vi "Resize and Align.vi"(9 "number of channels":i32, 10 "Refnums for Resizing and Alignment":T4, 11 "State in":T1={"Graph Visible Items"={"Plot Legend"=FALSE, "Scale Legend"=FALSE, "Graph Palette"=FALSE, "Cursor Legend"=FALSE, "X Scrollbar"=FALSE}, "View Table"=FALSE, "Table Visible Items"={"Vertical Scrollbar"=FALSE, "Horizontal Scrollbar"=FALSE, "Row Headers"=FALSE, "Column Headers"=FALSE, "Vertical Lines"=FALSE, "Horizontal Lines"=FALSE}, "Header Font"={"Font Name"="", "Size"=0, "Bold"=FALSE, "Italic"=FALSE, "Underline"=FALSE, "Strikeout"=FALSE, "Color"=0}, "Cell Font"={"Font Name"="", "Size"=0, "Bold"=FALSE, "Italic"=FALSE, "Underline"=FALSE, "Strikeout"=FALSE, "Color"=0}, "Description and Tip..."={"Description"="", "Tip"=""}, "Moveable Splitter Position"=0, "Measurement Cursor Configuration"={"relative to t0"={"enable relative time"=FALSE, "Relative times (DT)"=[], "color"=0}, "range"={"enable range"=FALSE, "T1"=0.0, "T2"=0.0, "Fixed interval (T2-T1)"=0.0, "T1 color"=0, "T2 color"=0, "enable shading"=FALSE}, "periodic"={"enable periodic"=FALSE, "First event (E1)"=0.0, "Number events (Ei)"=0, "Event spacing (s)"=0.0, "First color"=0, "Events color"=0}, "absolute timestamp"={"enable absolute"=FALSE, "Timestamps (TS)"=[], "color"=0}}, "X Increment"=0.0, "X Scale"={"Label Visible"=FALSE, "Label Text"="", "Time Mode"=enum."Relative", "Format String"=""}, "Y Scale"={"Label Visible"=FALSE, "Label Text"="", "Scaling"=enum."Engineering Units", "Format String"=""}, "Colors"={"background"=16777215, "major grid"=8355711, "minor grid"=12632256, "font"=0}, "Cursors"={"List"=[], "Tags"=[]}, "Plots"=[], "Plot Color Wheel"=[3381759, 32768, 982784, 4375295, 13827953, 13457919, 16757522, 4343295, 16728758, 12095254], "registered user events"=variant} caption="State") -> (0 "error out":errorcluster, 3 "State out":T1={"Graph Visible Items"={"Plot Legend"=FALSE, "Scale Legend"=FALSE, "Graph Palette"=FALSE, "Cursor Legend"=FALSE, "X Scrollbar"=FALSE}, "View Table"=FALSE, "Table Visible Items"={"Vertical Scrollbar"=FALSE, "Horizontal Scrollbar"=FALSE, "Row Headers"=FALSE, "Column Headers"=FALSE, "Vertical Lines"=FALSE, "Horizontal Lines"=FALSE}, "Header Font"={"Font Name"="", "Size"=0, "Bold"=FALSE, "Italic"=FALSE, "Underline"=FALSE, "Strikeout"=FALSE, "Color"=0}, "Cell Font"={"Font Name"="", "Size"=0, "Bold"=FALSE, "Italic"=FALSE, "Underline"=FALSE, "Strikeout"=FALSE, "Color"=0}, "Description and Tip..."={"Description"="", "Tip"=""}, "Moveable Splitter Position"=0, "Measurement Cursor Configuration"={"relative to t0"={"enable relative time"=FALSE, "Relative times (DT)"=[], "color"=0}, "range"={"enable range"=FALSE, "T1"=0.0, "T2"=0.0, "Fixed interval (T2-T1)"=0.0, "T1 color"=0, "T2 color"=0, "enable shading"=FALSE}, "periodic"={"enable periodic"=FALSE, "First event (E1)"=0.0, "Number events (Ei)"=0, "Event spacing (s)"=0.0, "First color"=0, "Events color"=0}, "absolute timestamp"={"enable absolute"=FALSE, "Timestamps (TS)"=[], "color"=0}}, "X Increment"=0.0, "X Scale"={"Label Visible"=FALSE, "Label Text"="", "Time Mode"=enum."Relative", "Format String"=""}, "Y Scale"={"Label Visible"=FALSE, "Label Text"="", "Scaling"=enum."Engineering Units", "Format String"=""}, "Colors"={"background"=16777215, "major grid"=8355711, "minor grid"=12632256, "font"=0}, "Cursors"={"List"=[], "Tags"=[]}, "Plots"=[], "Plot Color Wheel"=[3381759, 32768, 982784, 4375295, 13827953, 13457919, 16757522, 4343295, 16728758, 12095254], "registered user events"=variant} caption="State")   [LabVIEW 2017, in "Waveforms with Cursors.xctl"]
doc: "Based on moveable splitter position and pane sizes, resize the graph and table and align table with plot area."
uses:
  <vilib>/addons/_XControls/Waveforms with Cursors/Waveforms with Cursors.xctl
  <vilib>/addons/_XControls/Waveforms with Cursors/Controls/Refnums Typedef.ctl
  <vilib>/addons/_XControls/Waveforms with Cursors/Controls/State.ctl
  <vilib>/Utility/miscctls.llb/LVFontTypeDef.ctl
  <vilib>/addons/_XControls/Waveforms with Cursors/Controls/Waveform Cursor Configuration.ctl
  <vilib>/Utility/miscctls.llb/LVPositionTypeDef.ctl
  <vilib>/Utility/miscctls.llb/LVRowAndColumnTypeDef.ctl
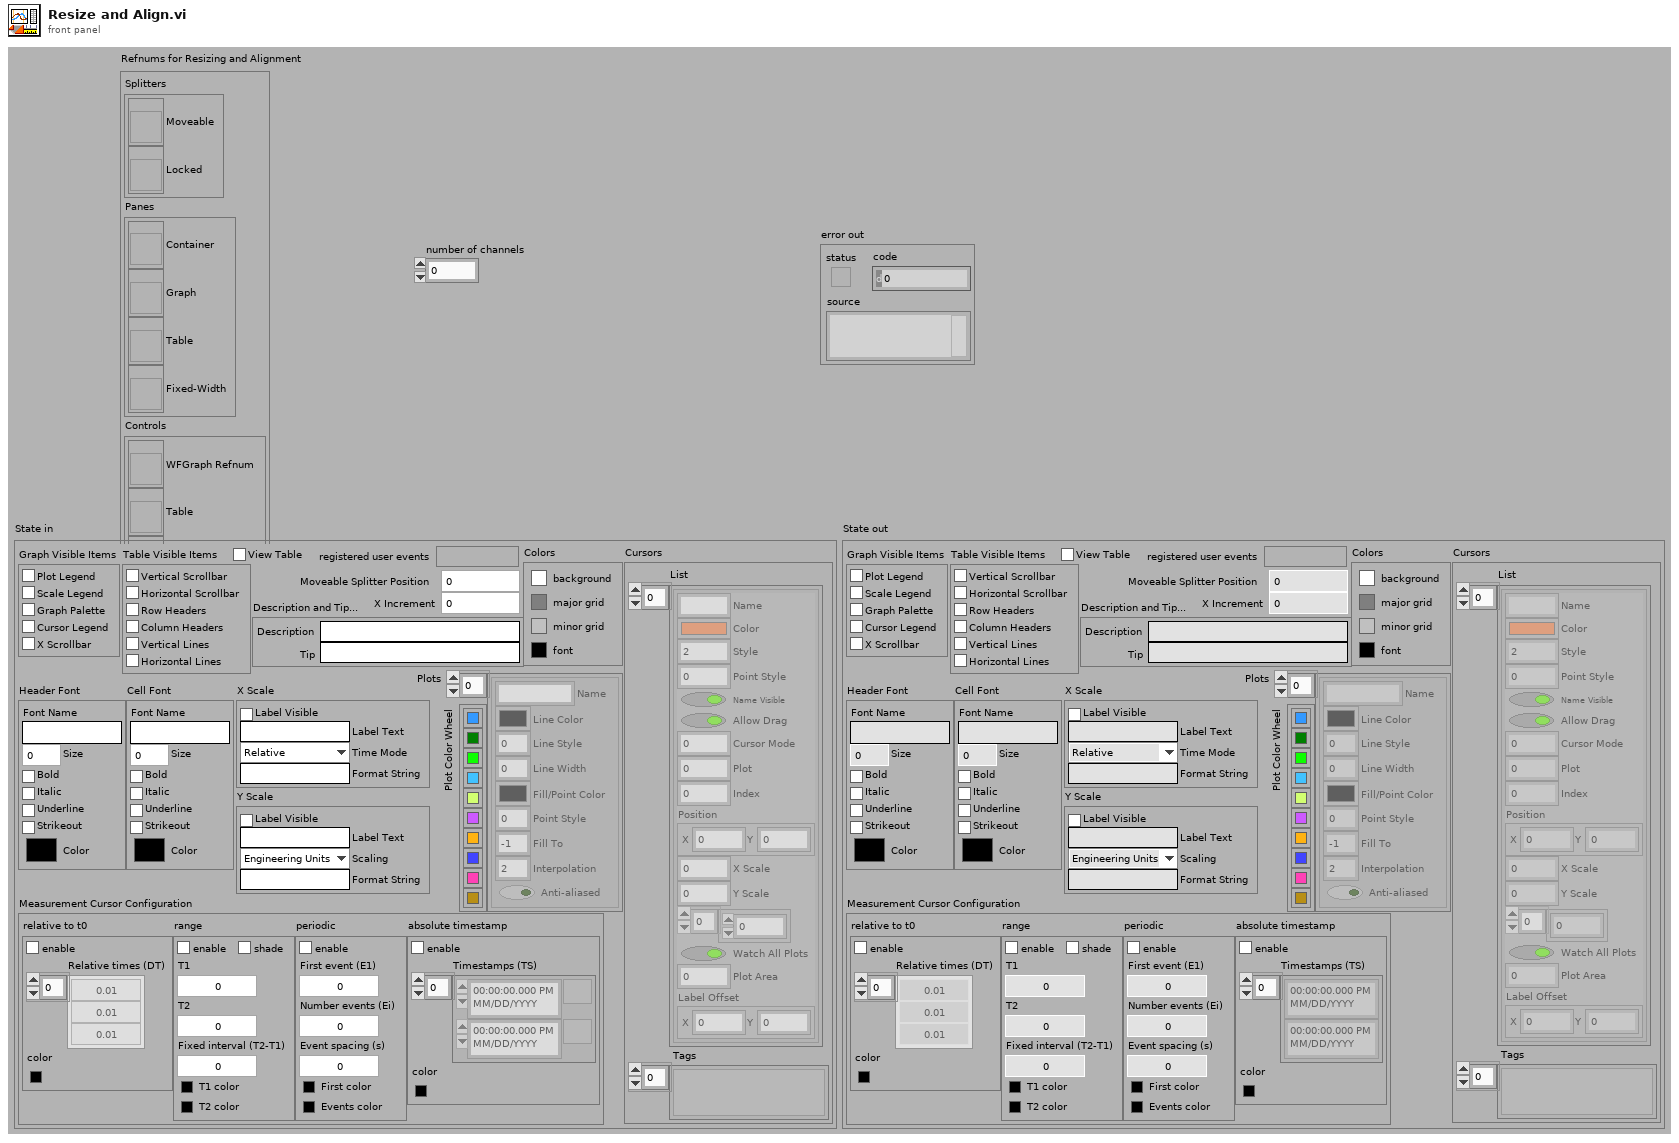
[diagram p1: front panel]
types:
  T1 = typedef "Waveforms with Cursors.xctl/State.ctl" = cluster{"Graph Visible Items":cluster{"Plot Legend":bool, "Scale Legend":bool, "Graph Palette":bool, "Cursor Legend":bool, "X Scrollbar":bool}, "View Table":bool, "Table Visible Items":cluster{"Vertical Scrollbar":bool, "Horizontal Scrollbar":bool, "Row Headers":bool, "Column Headers":bool, "Vertical Lines":bool, "Horizontal Lines":bool}, "Header Font":T2, "Cell Font":T2, "Description and Tip...":cluster{"Description":string, "Tip":string}, "Moveable Splitter Position":i32, "Measurement Cursor Configuration":T3, "X Increment":dbl, "X Scale":cluster{"Label Visible":bool, "Label Text":string, "Time Mode":enum16{"Relative", "Absolute"}, "Format String":string}, "Y Scale":cluster{"Label Visible":bool, "Label Text":string, "Scaling":enum16{"Engineering Units", "Voltage"}, "Format String":string}, "Colors":cluster{"background":u32, "major grid":u32, "minor grid":u32, "font":u32}, "Cursors":cluster{"List":cluster{"Name":string, "Color":u32, "Style":i32, "Point Style":u8, "Name Visible":bool, "Allow Drag":bool, "Cursor Mode":u32, "Plot":i32, "Index":i32, "Position":cluster{"X":dbl, "Y":dbl}, "X Scale":u32, "Y Scale":u32, "Watch Plots":i32[], "Watch All Plots":bool, "Plot Area":i32, "Label Offset":cluster{"X":dbl, "Y":dbl}}[], "Tags":variant[]}, "Plots":cluster{"Name":string, "Line Color":u32, "Line Style":u8, "Line Width":u8, "Fill/Point Color":u32, "Point Style":u8, "Fill To":i16, "Interpolation":u8, "Anti-aliased":bool}[], "Plot Color Wheel":u32[], "registered user events":variant}
  T2 = typedef "LVFontTypeDef.ctl" = cluster{"Font Name":string, "Size":u16, "Bold":bool, "Italic":bool, "Underline":bool, "Strikeout":bool, "Color":u32}
  T3 = typedef "Waveforms with Cursors.xctl/Waveform Cursor Configuration.ctl" = cluster{"relative to t0":cluster{"enable relative time":bool, "Relative times (DT)":dbl[], "color":u32}, "range":cluster{"enable range":bool, "T1":dbl, "T2":dbl, "Fixed interval (T2-T1)":dbl, "T1 color":u32, "T2 color":u32, "enable shading":bool}, "periodic":cluster{"enable periodic":bool, "First event (E1)":dbl, "Number events (Ei)":i32, "Event spacing (s)":dbl, "First color":u32, "Events color":u32}, "absolute timestamp":cluster{"enable absolute":bool, "Timestamps (TS)":timestamp[], "color":u32}}
  T4 = typedef "Waveforms with Cursors.xctl/Refnums Typedef.ctl" = cluster{"Splitters":cluster{"Moveable":refnum<vi>, "Locked":refnum<vi>}, "Panes":cluster{"Container":refnum<vi>, "Graph":refnum<vi>, "Table":refnum<vi>, "Fixed-Width":refnum<vi>}, "Controls":cluster{"WFGraph Refnum":refnum<vi>, "Table":refnum<vi>, "View Table":refnum<vi>, "Focus Boolean":refnum<vi>, "Plot Names":refnum<vi>}}
  T5 = typedef "LVPositionTypeDef.ctl" = cluster{"Left":i32, "Top":i32}
  T6 = typedef "LVRectTypeDef.ctl" = cluster{"Left":i16, "Top":i16, "Right":i16, "Bottom":i16}
  T7 = typedef "LVRowAndColumnTypeDef.ctl" = cluster{"Row":i32, "Column":i32}
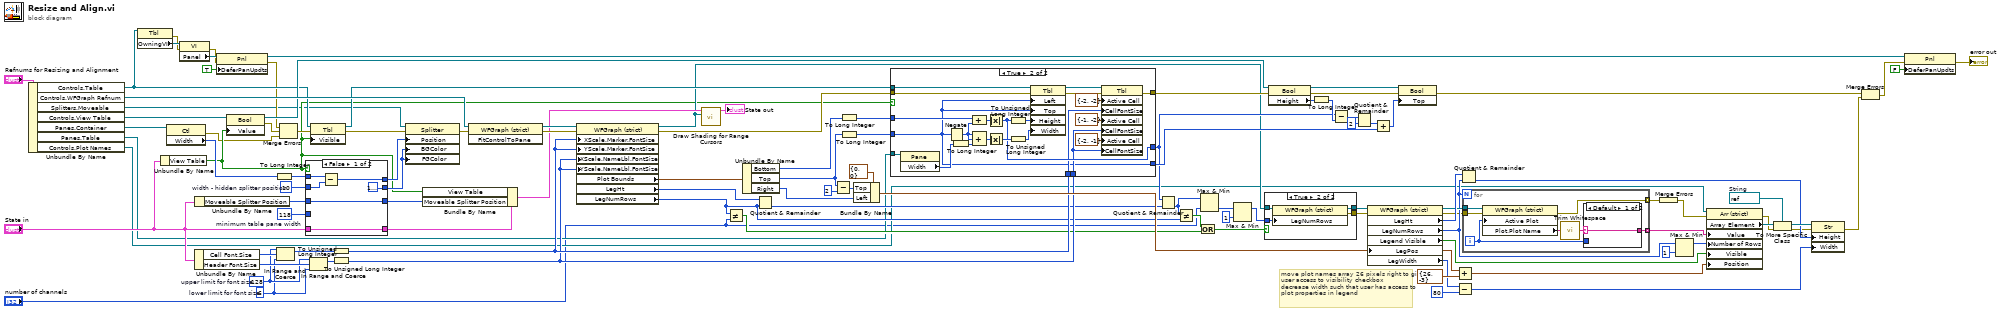
[diagram p0: block diagram]
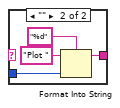
[diagram p3: hidden frame]
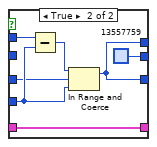
[diagram p4: hidden frame]
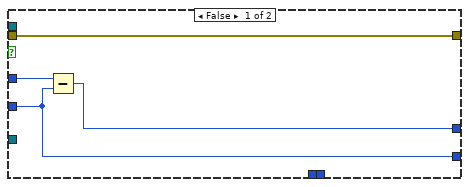
[diagram p5: hidden frame]
diagram:
  w2 = 10  # width - hidden splitter position
  w67 = u16 128  # upper limit for font size
  w66 = u16 6  # lower limit for font size
  w85 = refnum<vi> refnum  # String
  w86 = 118  # minimum table pane width
  # "move plot names array 26 pixels right to give user access to visibility checkbox\ndecrease width such that user has access to plot properties in legend"
  n1 = Unbundle By Name("Refnums for Resizing and Alignment") -> ("Controls.Table"=w22:refnum<vi>, "Controls.WFGraph Refnum"=w103:refnum<vi>, "Splitters.Moveable"=w6:refnum<vi>, "Controls.View Table"=w23:refnum<vi>, "Panes.Container"=w9:refnum<vi>, "Panes.Table"=w8:refnum<vi>, "Controls.Plot Names"=w7:refnum<vi>)
  n2 = property class="Tbl"(reference=w22) -> (error out=w31:errorcluster, "OwningVI"=w50:refnum<vi>)  [unwired: 1 in, 1 out]
  n3 = Unbundle By Name("State in") -> ("View Table"=w10:bool)
  n4 = property class="Ctl"(reference=w9) -> (error out=w4:errorcluster, "Width"=w102:u32)  [unwired: 1 in, 1 out]
  n5 = property class="VI"(reference=w50, error in=w31) -> (error out=w30:errorcluster, "Panel"=w49:refnum<vi>)  [unwired: 1 out]
  n6 = Unbundle By Name("State in") -> ("Cell Font.Size"=w68:u16, "Header Font.Size"=w69:u16)
  n7 = Unbundle By Name("State in") -> ("Moveable Splitter Position"=w99:i32)
  n8 = property class="Pnl"(reference=w49, error in=w30, "DeferPanUpdts"=TRUE ("Defer Panel Updates")) -> (reference out=w42:refnum<vi>, error out=w16:errorcluster)
  n9 = property class="Bool"(reference=w23, "Value"=w10) -> (reference out=w98:refnum<vi>, error out=w5:errorcluster)  [unwired: 1 in]
  n10 = To Long Integer(number=w102) -> (32bit integer=w3:i32)
  n11 = In Range and Coerce(upper limit=w67, x=w68, lower limit=w66) -> (coerced(x)=w63:u16)  [unwired: 1 out]
  n12 = Merge Errors(w16, w5, w4) -> (w17:errorcluster)
  n13 = case shown="False" w10 {
    tunnel: w3 -> [w110 w118]
    tunnel: [w108 w119] -> w101
    tunnel: [u32 16777216 ("Color Box") u32 13557759 ("Color Box")] -> w100
    tunnel: [w112 w119] -> w87
    tunnel: w99 -> [w112 w114]
    tunnel: w86 -> [_ w117]
    tunnel: "State in" -> [w111 w116]
    tunnel: [w111 w116] -> w15
    tunnel: w2 -> [w109 _]
    frame False {
      n14 = Subtract(x=w110, y=w109) -> (x-y=w108:i32)
    }
    frame True {
      n15 = Subtract(x=w118, y=w117) -> (x-y=w120:i32)
      n16 = In Range and Coerce(upper limit=w120, x=w114, lower limit=w117) -> (coerced(x)=w119:i32)  [unwired: 1 out]
    }
  }
  n17 = In Range and Coerce(upper limit=w67, x=w69, lower limit=w66) -> (coerced(x)=w62:u16)  [unwired: 1 out]
  n18 = property class="Tbl"(reference=w22, error in=w17, "Visible"=w10) -> (reference out=w64:refnum<vi>, error out=w65:errorcluster)
  n19 = To Unsigned Long Integer(number=w63) -> (unsigned 32bit integer=w61:u32)
  n20 = To Unsigned Long Integer(number=w62) -> (unsigned 32bit integer=w60:u32)
  n21 = property class="Splitter"(reference=w6, error in=w65, "Position"=w101, "BGColor"=w100, "FGColor"=w100) -> (error out=w105:errorcluster)  [unwired: 1 out]
  n22 = Bundle By Name(cluster=w15, "View Table"=w10, "Moveable Splitter Position"=w87) -> (w13:T1)
  n23 = invoke class="WFGraph (strict)" method="FitControlToPane"(reference=w103, error in=w105) -> (reference out=w107:refnum<vi>, error out=w106:errorcluster)  [unwired: 1 in, 1 out]
  n24 = property class="WFGraph (strict)"(reference=w107, error in=w106, "XScale.Marker.FontSize"=w61, "YScale.Marker.FontSize"=w61, "XScale.NameLbl.FontSize"=w60, "YScale.NameLbl.FontSize"=w60) -> (reference out=w12:refnum<vi>, error out=w104:errorcluster, "Plot Bounds"=w56:T6, "LegHt"=w29:u32, "LegNumRows"=w25:u32)
  n25 = call <vilib>:"Draw Shading for Range Cursors.vi"("WaveformGraph"=w12, "Display State In"=w13) -> ("Display State Out"=→"State out":T1)  [unwired: 9 in]
  n26 = Not Equal?(x=w25, y="number of channels") -> (x != y?=w32:bool)
  n27 = Unbundle By Name(w56) -> ("Bottom"=w55:i16, "Top"=w77:i16, "Right"=w78:i16)
  n28 = Quotient & Remainder(x=w29, y=w25) -> (floor(x/y)=w27:u32)  [unwired: 1 out]
  n29 = Subtract(x=w77, y=i16 2) -> (x-y=w76:i16)
  n30 = To Long Integer(number=w55) -> (32bit integer=w88:i32)
  n31 = To Long Integer(number=w77) -> (32bit integer=w59:i32)
  n32 = Bundle By Name(cluster=T5 {"Left"=0, "Top"=0} ("Legend:Position"), "Top"=w76, "Left"=w78) -> (w70:T5)
  n33 = case shown="True" w10 {
    tunnel: w64 -> [_ w146]
    tunnel: w59 -> [w121 w125]
    tunnel: w88 -> [w123 w145]
    tunnel: w8 -> [_ w143]
    tunnel: w104 -> [w124 w140]
    tunnel: [w124 w126] -> w95
    tunnel: [w122 w132] -> w26
    tunnel: w61 -> [_ w130]
    tunnel: w60 -> [_ w127]
    tunnel: [w121 w125] -> w28
    frame False {
      n34 = Subtract(x=w123, y=w121) -> (x-y=w122:i32)
    }
    frame True {
      n35 = property class="Pane"(reference=w143) -> ("Width"=w142:u32)  [unwired: 1 in, 2 out]
      n36 = Negate(x=w125) -> (-x=w137:i32)
      n37 = To Long Integer(number=w142) -> (32bit integer=w138:i32)
      n38 = Compound Arithmetic op=ADD(w145, w137) -> (w144:i32)
      n39 = Compound Arithmetic op=ADD(w137, w137, w138) -> (w141:i32)
      n40 = Absolute Value(x=w144) -> (abs(x)=w132:i32)
      n41 = Absolute Value(x=w141) -> (abs(x)=w135:i32)
      n42 = To Unsigned Long Integer(number=w132) -> (unsigned 32bit integer=w139:u32)
      n43 = To Unsigned Long Integer(number=w135) -> (unsigned 32bit integer=w136:u32)
      n44 = property class="Tbl"(reference=w146, error in=w140, "Left"=w125, "Top"=w125, "Height"=w139, "Width"=w136) -> (reference out=w134:refnum<vi>, error out=w133:errorcluster)
      n45 = property class="Tbl"(reference=w134, error in=w133, "Active Cell"=T7 {"Row"=-2, "Column"=-2} ("Active Cell:Active Cell"), "CellFontSize"=w130, "Active Cell"=T7 {"Row"=-1, "Column"=-2} ("Active Cell:Active Cell"), "CellFontSize"=w127, "Active Cell"=T7 {"Row"=-2, "Column"=-1} ("Active Cell:Active Cell"), "CellFontSize"=w127) -> (error out=w126:errorcluster)  [unwired: 1 out]
    }
  }
  n46 = Quotient & Remainder(x=w26, y=w27) -> (floor(x/y)=w19:u32)  [unwired: 1 out]
  n47 = Not Equal?(x=w19, y=w25) -> (x != y?=w24:bool)
  n48 = Or(x=w24, y=w32) -> (x .or. y?=w33:bool)
  n49 = Max & Min(x=w19, y="number of channels") -> (min(x,y)=w20:u32)  [unwired: 1 out]
  n50 = Max & Min(x=w20, y=u32 1 ("lower limit")) -> (max(x,y)=w18:u32)  [unwired: 1 out]
  n51 = case shown="True" w33 {
    tunnel: w12 -> [w147 w151]
    tunnel: [w147 w150] -> w40
    tunnel: w18 -> [_ w149]
    tunnel: [_ w148] -> w39
    frame False {
    }
    frame True {
      n52 = property on="Property Node" class="WFGraph (strict)"(reference=w151, "LegNumRows"=w149) -> (reference out=w150:refnum<vi>, error out=w148:errorcluster)  [unwired: 1 in]
    }
  }
  n53 = property class="Bool"(reference=w98, error in=w95) -> (reference out=w97:refnum<vi>, error out=w94:errorcluster, "Height"=w96:u32)
  n54 = To Long Integer(number=w96) -> (32bit integer=w93:i32)
  n55 = Subtract(x=w26, y=w93) -> (x-y=w92:i32)
  n56 = Quotient & Remainder(x=w92, y=2) -> (floor(x/y)=w90:i32)  [unwired: 1 out]
  n57 = property on="Property Node" class="WFGraph (strict)"(reference=w40, error in=w39, "LegPos"=w70) -> (reference out=w53:refnum<vi>, error out=w38:errorcluster, "LegHt"=w57:u32, "LegNumRows"=w41:u32, "Legend Visible"=w58:bool, "LegWidth"=w71:u32)
  n58 = Add(x=w90, y=w28) -> (x+y=w89:i32)
  n59 = property class="Bool"(reference=w97, error in=w94, "Top"=w89) -> (error out=w46:errorcluster)  [unwired: 1 out]
  n60 = Add(x=w70, y=T5 {"Left"=26, "Top"=-3}) -> (x+y=w81:T5)
  n61 = Subtract(x=w71, y=u32 80) -> (x-y=w72:u32)
  n62 = Quotient & Remainder(x=w57, y=w41) -> (floor(x/y)=w75:u32)  [unwired: 1 out]
  n63 = for {
    N: w41 -> [_]
    tunnel: [w158] -> w73 mode=indexing
    tunnel: w53 -> [w157]
    tunnel: w38 -> [w153]
    tunnel: [w152] -> w37 mode=indexing
    i -> [w154]
    n64 = property on="Property Node" class="WFGraph (strict)"(reference=w157, error in=w153, "Active Plot"=w154) -> (error out=w152:errorcluster, "Plot.Plot Name"=w156:string)  [unwired: 1 out]
    n65 = call <vilib>:"Trim Whitespace.vi"("string"=w156) -> ("trimmed string"=w155:string)  [unwired: 1 in]
    n66 = case shown="Default" w155 {
      selector: w155 -> [w159 _]
      tunnel: w154 -> [_ w163]
      tunnel: [w159 w160] -> w158
      frame Default {
      }
      frame "" {
        n67 = Format Into String(format string="%d", initial string="Plot ", w163) -> (resulting string=w160:string)  [unwired: 1 in, 1 out]
      }
    }
  }
  n68 = Merge Errors(w37) -> (w36:errorcluster)
  n69 = Max & Min(x=w41, y=u32 1 ("lower limit")) -> (max(x,y)=w52:u32)  [unwired: 1 out]
  n70 = property on="Property Node" class="Arr (strict)"(reference=w7, error in=w36, "Value"=w73, "Number of Rows"=w52, "Visible"=w58, "Position"=w81) -> (error out=w35:errorcluster, "Array Element"=w74:refnum<vi>)  [unwired: 1 out]
  n71 = To More Specific Class(target class=w85, reference=w74, error in=w35) -> (specific class reference=w84:refnum<vi>, error out=w34:errorcluster)
  n72 = property class="Str"(reference=w84, error in=w34, "Height"=w75, "Width"=w72) -> (error out=w45:errorcluster)  [unwired: 1 out]
  n73 = Merge Errors(w46, w45) -> (w44:errorcluster)
  n74 = property class="Pnl"(reference=w42, error in=w44, "DeferPanUpdts"=FALSE ("Defer Panel Updates")) -> (error out=→"error out":errorcluster)  [unwired: 1 out]
